vi "SetRate.vi"(2 "error in (no error)":errorcluster, 3 "rate":dbl, 4 "Task ID":u32) -> (0 "error out":errorcluster, 1 "Task ID":u32)   [LabVIEW 2015]
uses:
  Windows/System32/AdvLvDaq.dll
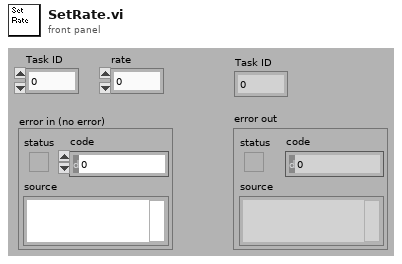
[diagram p1: front panel]
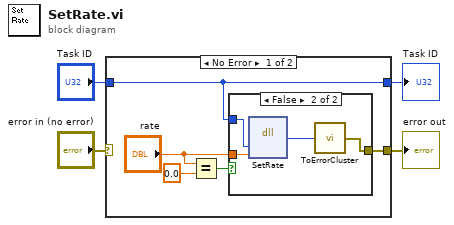
[diagram p0: block diagram]
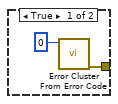
[diagram p2: hidden frame]
diagram:
  n1 = case shown="No Error" "error in (no error)" {
    selector: "error in (no error)" -> [_ w17]
    tunnel: [w9 w17] -> w3
    tunnel: "Task ID" -> [w8 w16]
    tunnel: [w8 w16] -> w1
    frame No Error {
      n2 = Equal?(x="rate", y=0.0) -> (x = y?=w7:bool)
      n3 = case shown="False" w7 {
        tunnel: [w11 w14] -> w9
        tunnel: w8 -> [_ w13]
        tunnel: "rate" -> [_ w12]
        frame True {
          n4 = call <vilib>:"Error Cluster From Error Code.vi"("error code (0)"=0) -> ("error out"=w11:errorcluster)  [unwired: 2 in, 6 out]
        }
        frame False {
          n5 = dll-call lib="C:/Windows/System32/AdvLvDaq.dll" fn="SetRate"("taskId"=w13, "rate"=w12) -> ("return type"=w15:i32)  [unwired: 5 in, 2 out]
          n6 = call "ToErrorCluster.vi"("error code"=w15) -> ("error out"=w14:errorcluster)
        }
      }
    }
    frame Error {
    }
  }
  "error out" <- w3
  "Task ID" <- w1
